vi "Defer Panel Update - FALSE.vi"(8 "error in (no error)":errorcluster, 11 "reference":refnum<vi>) -> (0 "error out":errorcluster, 3 "reference out":refnum<vi>)   [LabVIEW 2019, in "UI Tools.lvlib"]
doc: "Defer Panel Update - FALSE."
uses:
  UI Tools.lvlib
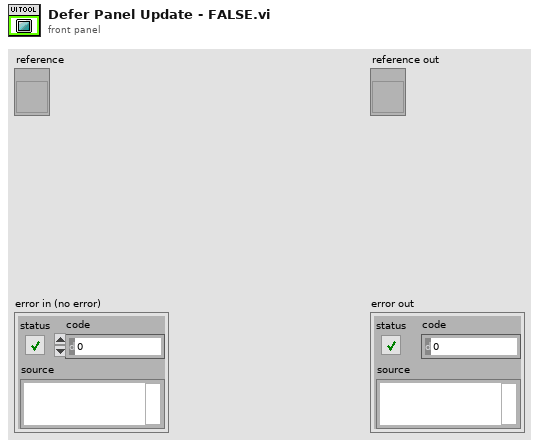
[diagram p1: front panel]
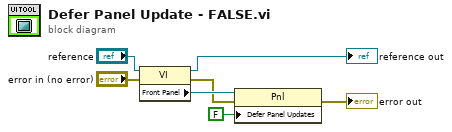
[diagram p0: block diagram]
diagram:
  n1 = property class="VI"(reference="reference", error in="error in (no error)") -> (reference out=→"reference out":refnum<vi>, error out=w2:errorcluster, "Front Panel"=w3:refnum<vi>)
  n2 = property class="Pnl"(reference=w3, error in=w2, "Defer Panel Updates"=FALSE) -> (error out=→"error out":errorcluster)  [unwired: 1 out]
